vi "GetValueFromSettingsFile.vi"(8 "error in (no error)":errorcluster caption="에러 입력(에러 없음)", 11 "init 파일 경로":string) -> (0 "error out":errorcluster caption="에러 출력", 3 "출력 클러스터":T1)   [LabVIEW 2018]
uses:
  <vilib>/Utility/config.llb/NI_LVConfig.lvlib
  <vilib>/Utility/config.llb/Read Key (String).vi
  SettingsFileData.ctl
  <vilib>/Utility/config.llb/Read Key (Path).vi
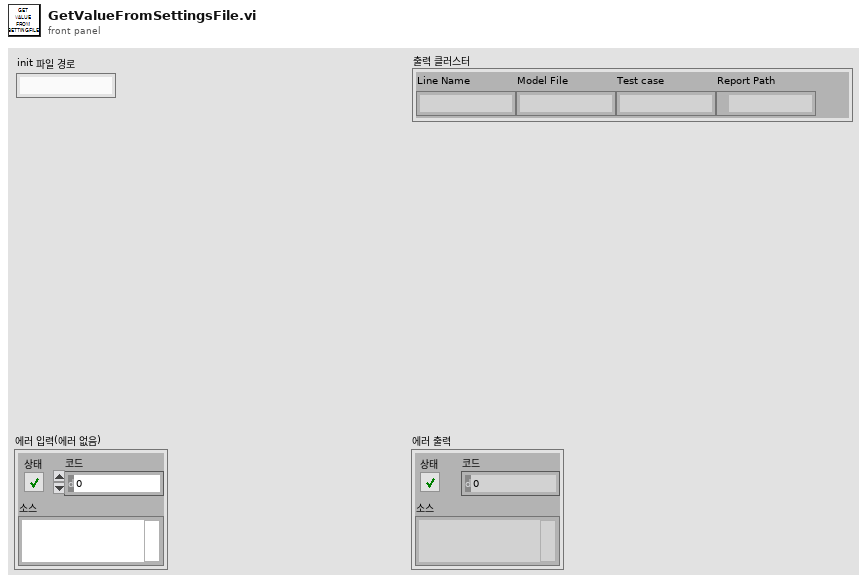
[diagram p1: front panel]
types:
  T1 = typedef "SettingsFileData.ctl" = cluster{"Line Name":string, "Model File":string, "Test case":string, "Report Path":path}
  T2 = typedef "NI_LVConfig.lvlib/Config Data RefNum.ctl" = refnum<k1>
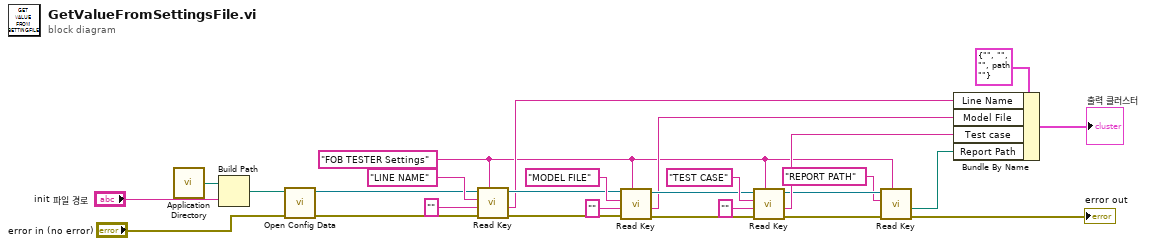
[diagram p0: block diagram]
diagram:
  w3 = "FOB TESTER Settings" ("section")
  n1 = call <vilib>:"Application Directory.vi"() -> ("Application Directory"=w27:path)
  n2 = Build Path(base path=w27, name or relative path="init 파일 경로") -> (appended path=w26:path)
  n3 = call <vilib>:"Open Config Data.vi"("error in (no error)"="error in (no error)", "configuration file path"=w26) -> ("error out"=w17:errorcluster, "refnum"=w16:T2)  [unwired: 7 in, 1 out]
  n4 = call-poly <vilib>:"Read Key.vi"("section"=w3, "error in (no error)"=w17, "default value"="", "key"="LINE NAME", "refnum"=w16) -> ("error out"=w19:errorcluster, "value"=w11:string, "refnum out"=w22:T2)  [unwired: 3 in, 1 out]
  n5 = call-poly <vilib>:"Read Key.vi"("section"=w3, "error in (no error)"=w19, "default value"="", "key"="MODEL FILE", "refnum"=w22) -> ("error out"=w13:errorcluster, "value"=w10:string, "refnum out"=w12:T2)  [unwired: 3 in, 1 out]
  n6 = call-poly <vilib>:"Read Key.vi"("section"=w3, "error in (no error)"=w13, "default value"="", "key"="TEST CASE", "refnum"=w12) -> ("error out"=w6:errorcluster, "value"=w9:string, "refnum out"=w4:T2)  [unwired: 3 in, 1 out]
  n7 = call-poly <vilib>:"Read Key.vi"("section"=w3, "error in (no error)"=w6, "key"="REPORT PATH", "refnum"=w4) -> ("error out"=→"error out":errorcluster, "value"=w1:path)  [unwired: 4 in, 2 out]
  n8 = Bundle By Name(cluster=T1 {"Line Name"="", "Model File"="", "Test case"="", "Report Path"=path ""} ("SettingData"), "Line Name"=w11, "Model File"=w10, "Test case"=w9, "Report Path"=w1) -> (→"출력 클러스터":T1)
